vi "Determine Starting Trim.vi"(5 "Target_Trim":dbl=10.0 format="%#_6p", 7 "Initial_Trim_Meas":dbl=10.0 format="%#_6p", 10 "Trim_Deltas":string[](array[string])=["0", "1.01", "2.02", "3.03", "4.04", "5.05", "6.06", "7.11", "7.81", "8.53", "9.11", "9.71", "10.2", "10.75", "11.3", "11.96"], 11 "Trim_States":string[](array[string])=["0\n1\n2\n3\n4\n5\n6\n7\n8\n9\n10\n11\n12\n13\n14\n15\n", "1", "2", "3", "4", "5", "6", "7", "8", "9", "10", "11", "12", "13", "14", "15"]) -> (2 "Delta_Trim":dbl, 3 "Starting_Trim":u8)   [LabVIEW 2013]
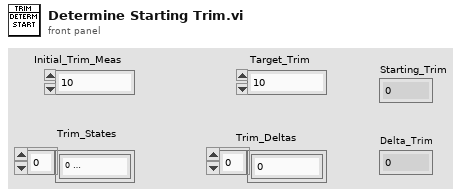
[diagram p1: front panel]
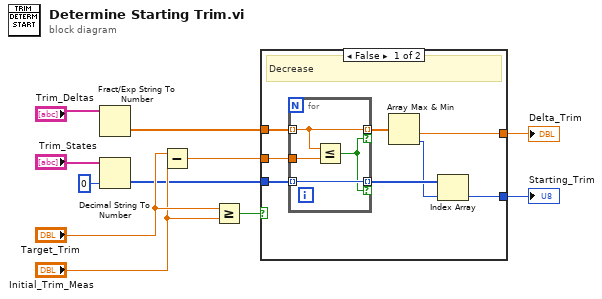
[diagram p0: block diagram]
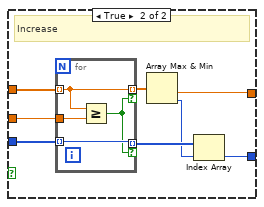
[diagram p2: hidden frame]
diagram:
  n1 = Fract/Exp String To Number(string="Trim_Deltas") -> (number=w6:dbl[])  [unwired: 3 in, 1 out]
  n2 = Decimal String To Number(string="Trim_States", default (0L)=u8 0 ("element")) -> (number=w3:u8[])  [unwired: 1 in, 1 out]
  n3 = Subtract(x="Target_Trim", y="Initial_Trim_Meas") -> (x-y=w7:dbl)
  n4 = Greater Or Equal?(x="Target_Trim", y="Initial_Trim_Meas") -> (x >= y?=w8:bool)
  n5 = case shown="False" w8 {
    tunnel: w7 -> [w18 w30]
    tunnel: w6 -> [w19 w31]
    tunnel: w3 -> [w16 w28]
    tunnel: [w13 w25] -> w1
    tunnel: [w12 w24] -> w2
    frame False {
      # "Decrease"
      n6 = for {
        tunnel: w19 -> [w22] mode=indexing
        tunnel: w18 -> [w23]
        tunnel: [w22] -> w17 mode=indexing if=w20
        tunnel: w16 -> [w21] mode=indexing
        tunnel: [w21] -> w15 mode=indexing if=w20
        n7 = Less Or Equal?(x=w22, y=w23) -> (x <= y?=w20:bool)
      }
      n8 = Array Max & Min(array=w17) -> (min value=w12:dbl, min index (indices)=w14:i32)  [unwired: 2 out]
      n9 = Index Array(array=w15, index=w14) -> (element=w13:u8)
    }
    frame True {
      # "Increase"
      n10 = for {
        tunnel: w31 -> [w34] mode=indexing
        tunnel: w30 -> [w35]
        tunnel: [w34] -> w29 mode=indexing if=w32
        tunnel: w28 -> [w33] mode=indexing
        tunnel: [w33] -> w27 mode=indexing if=w32
        n11 = Greater Or Equal?(x=w34, y=w35) -> (x >= y?=w32:bool)
      }
      n12 = Array Max & Min(array=w29) -> (min value=w24:dbl, min index (indices)=w26:i32)  [unwired: 2 out]
      n13 = Index Array(array=w27, index=w26) -> (element=w25:u8)
    }
  }
  "Starting_Trim" <- w1
  "Delta_Trim" <- w2
